vi "SQL Connect.vi"(5 "SqlMapper Type":refnum<class "SqlMapper.lvclass">, 8 "error in (no error)":errorcluster, 10 "Connection String":string) -> (0 "error out":errorcluster, 3 "SQL Mapper":refnum<class "SqlMapper.lvclass">)   [LabVIEW 2020, in "ORM_DBC_Mssql.lvlib" / "DBC.lvclass"]
uses:
  DBC.lvclass
  <vilib>/Viviota/shared/ORM.lvlibp/ORM/SqlMapper/SqlMapper.lvclass
  DBC.lvclass/DBC.ctl
  C:/Program Files/National Instruments/LabVIEW 2020/vi.lib/Viviota/shared/ORM.lvlibp/ORM/DbConnection/DbConnection.lvclass
  C:/Viviota/Projects/R&D/LabVIEW_ORM/source/src/DbConnections/SQLConnection/DBC.lvclass
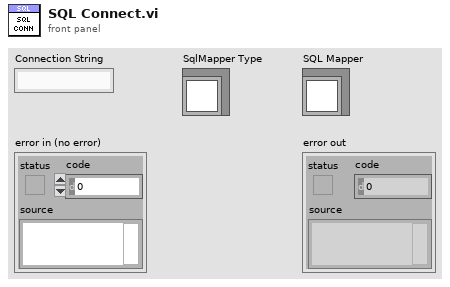
[diagram p1: front panel]
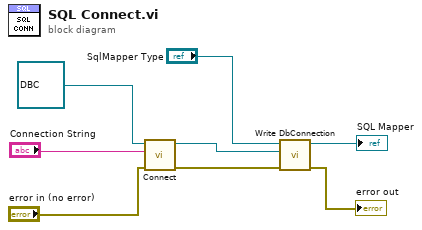
[diagram p0: block diagram]
diagram:
  n1 = call-dynamic "Connect.vi"("error in (no error)"="error in (no error)", "Connection String"="Connection String", "SQLConnection Type"=refnum<class "DBC.lvclass"> refnum) -> ("error out"=w5:errorcluster, "SQLConnection out"=w4:refnum<class "DBC.lvclass">)  [unwired: 7 in]
  n2 = call <vilib>:"Write DbConnection.vi"("error in (no error)"=w5, "Dapper.lvlib:DbConnection.lvclass"=w4, "SqlMapper in"="SqlMapper Type") -> ("error out"=→"error out":errorcluster, "SqlMapper out"=→"SQL Mapper":refnum<class "SqlMapper.lvclass">)  [unwired: 7 in]
